vi "Tokens to Object.vi"(8 "error in":errorcluster, 10 "starting index":i32, 11 "array w/ subset deleted":cluster{"Token Type":T1, "Token Value":string}[](array[cluster])) -> (0 "error out":errorcluster, 2 "next index":i32, 3 "JSON Object out":refnum<class "JSON Object.lvclass">)   [LabVIEW 2017, in "LVJSON.lvlib"]
uses:
  LVJSON.lvlib
  JSON Data Classes/JSON Object/JSON Object.lvclass
  C:/Users/tblair/Documents/Git Projects/LVJSON/JSON Data Classes/JSON Datatype/JSON Datatype.lvclass
  Token Types.ctl
  JSON Data Classes/JSON Array/JSON Array.lvclass
  JSON Data Classes/JSON Numeric/JSON Numeric.lvclass
  JSON Data Classes/JSON Boolean/JSON Boolean.lvclass
  JSON Data Classes/JSON Null/JSON Null.lvclass
  JSON Data Classes/JSON String/JSON String.lvclass
  JSON Data Classes/JSON Numeric/New JSON Numeric.vi
  JSON Data Classes/JSON Boolean/New JSON Boolean.vi
  JSON Data Classes/JSON Null/New JSON Null.vi
  JSON Data Classes/JSON String/New JSON String.vi
  JSON Data Classes/JSON Object/New JSON Object.vi
  JSON Data Classes/JSON Object/Insert Key Value Pair (Multi).vi
  JSON Data Classes/JSON Datatype/JSON Datatype.lvclass
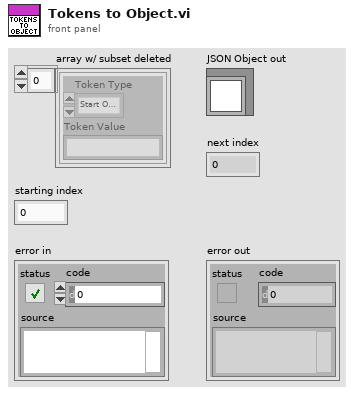
[diagram p1: front panel]
types:
  T1 = typedef "Token Types.ctl" = enum32{"Start Object", "End Object", "Start Array", "End Array", "Colon", "Comma", "Numeric", "true", "false", "null", "String"}
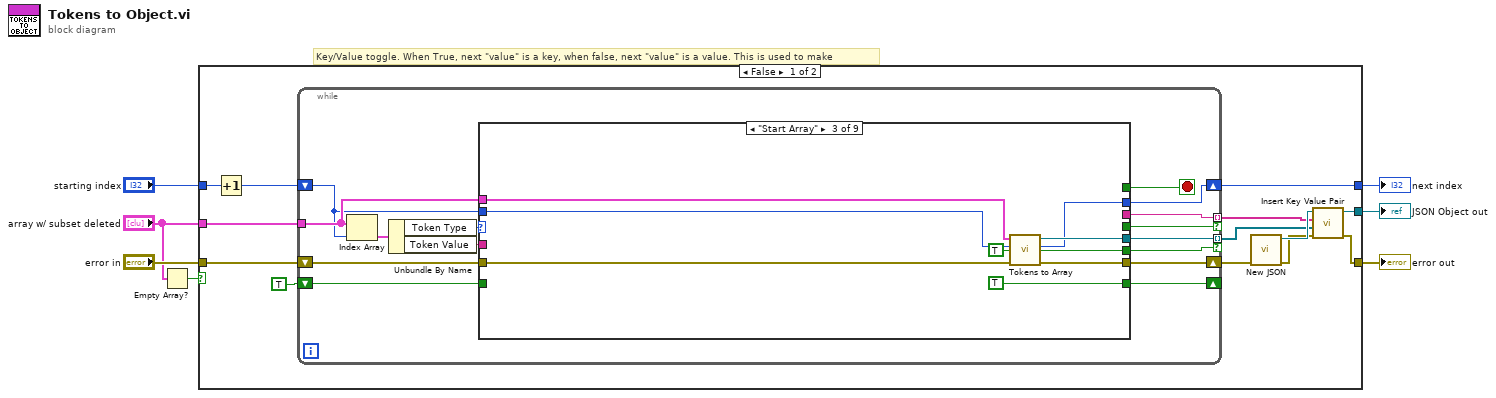
[diagram p0: block diagram]
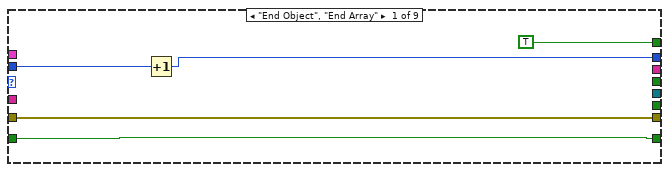
[diagram p2: hidden frame]
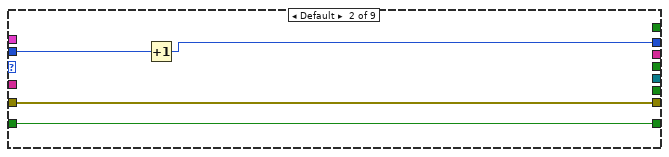
[diagram p3: hidden frame]
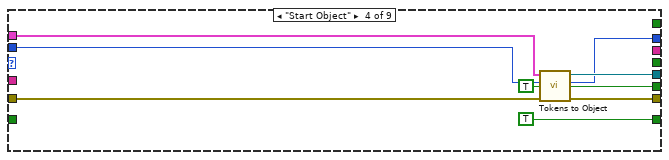
[diagram p4: hidden frame]
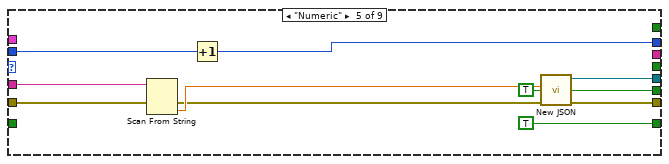
[diagram p5: hidden frame]
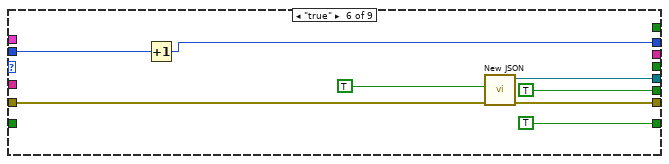
[diagram p6: hidden frame]
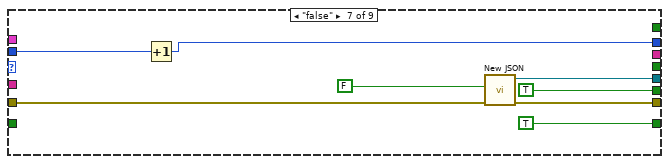
[diagram p7: hidden frame]
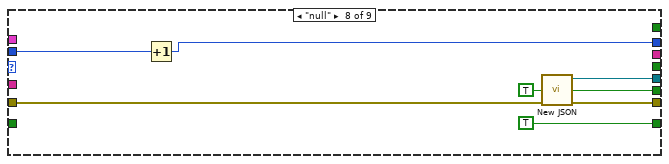
[diagram p8: hidden frame]
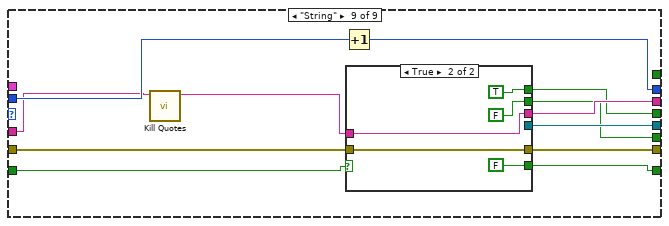
[diagram p9: hidden frame]
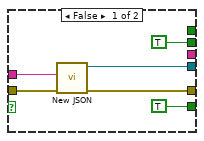
[diagram p10: hidden frame]
diagram:
  # "Key/Value toggle. When True, next \"value\" is a key, when false, next \"value\" is a value. This is used to make"
  n1 = Empty Array?(array="array w/ subset deleted") -> (empty?=w1:bool)
  n2 = case shown="False" w1 {
    tunnel: [w13 _] -> w7
    tunnel: "array w/ subset deleted" -> [w20 _]
    tunnel: "error in" -> [w19 w117]
    tunnel: [w8 w117] -> w5
    tunnel: [w16 w118] -> w4
    tunnel: "starting index" -> [w15 w118]
    frame False {
      n3 = Increment(x=w15) -> (x+1=w17:i32)
      n4 = while {
        tunnel: w20 -> [w28]
        tunnel: [w32] -> w12 mode=indexing if=w21
        shift-right: [w27] -> w16
        shift-left: w17 -> [w26]
        shift-right: [w29] -> w18
        shift-left: w19 -> [w30]
        shift-right: [w22] -> _
        shift-left: TRUE -> [w25]
        tunnel: [w24] -> w10 mode=indexing if=w23
        stop <- w33 stop-if-true
        n5 = Index Array(array=w28, index=w26) -> (element=w31:cluster{"Token Type":T1, "Token Value":string})
        n6 = Unbundle By Name(w31) -> ("Token Type"=w35:T1, "Token Value"=w34:string)
        n7 = case shown="\"Start Array\"" w35 {
          tunnel: w34 -> [_ _ _ _ w69 _ _ _ w94]
          tunnel: [TRUE _ _ _ _ _ _ _ _] -> w33
          tunnel: [_ _ w49 w57 w70 w77 w85 w93 w105] -> w32
          tunnel: [_ _ TRUE TRUE TRUE TRUE TRUE TRUE w97] -> w21
          tunnel: w30 -> [w40 w44 w52 w60 w66 w75 w83 w91 w96]
          tunnel: [w40 w44 w51 w59 w64 w74 w82 w90 w104] -> w29
          tunnel: w28 -> [_ _ w50 w58 _ _ _ _ _]
          tunnel: w26 -> [w39 w43 w46 w54 w63 w73 w81 w89 w103]
          tunnel: [w38 w42 w47 w55 w62 w72 w80 w88 w102] -> w27
          tunnel: w25 -> [w36 w41 _ _ _ _ _ _ w101]
          tunnel: [w36 w41 TRUE TRUE TRUE TRUE TRUE TRUE w98] -> w22
          tunnel: [_ _ _ _ _ _ _ _ w100] -> w24
          tunnel: [_ _ _ _ _ _ _ _ w99] -> w23
          frame "End Object", "End Array" {
            n8 = Increment(x=w39) -> (x+1=w38:i32)
          }
          frame Default {
            n9 = Increment(x=w43) -> (x+1=w42:i32)
          }
          frame "Start Array" {
            n10 = call "Tokens to Array.vi"("error in"=w52, "starting index"=w46, "array w/ subset deleted"=w50) -> ("error out"=w51:errorcluster, "next index"=w47:i32, "JSON Array out"=w49:refnum<class "JSON Array.lvclass">)  [unwired: 6 in]
          }
          frame "Start Object" {
            n11 = call "Tokens to Object.vi"("error in"=w60, "starting index"=w54, "array w/ subset deleted"=w58) -> ("error out"=w59:errorcluster, "next index"=w55:i32, "JSON Object out"=w57:refnum<class "JSON Object.lvclass">)  [unwired: 6 in]
          }
          frame "Numeric" {
            n12 = Scan From String(input string=w69, error in=w66) -> (error out=w65:errorcluster, output 1=w68:dbl)  [unwired: 3 in, 2 out]
            n13 = Increment(x=w63) -> (x+1=w62:i32)
            n14 = call-poly "New JSON.vi"("error in (no error)"=w65, "value"=w68) -> ("error out"=w64:errorcluster, "JSON String out"=w70:refnum<class "JSON Numeric.lvclass">)  [unwired: 8 in]
          }
          frame "true" {
            n15 = Increment(x=w73) -> (x+1=w72:i32)
            n16 = call-poly "New JSON.vi"("error in (no error)"=w75, "value"=TRUE) -> ("error out"=w74:errorcluster, "JSON String out"=w77:refnum<class "JSON Boolean.lvclass">)  [unwired: 8 in]
          }
          frame "false" {
            n17 = Increment(x=w81) -> (x+1=w80:i32)
            n18 = call-poly "New JSON.vi"("error in (no error)"=w83, "value"=FALSE) -> ("error out"=w82:errorcluster, "JSON String out"=w85:refnum<class "JSON Boolean.lvclass">)  [unwired: 8 in]
          }
          frame "null" {
            n19 = Increment(x=w89) -> (x+1=w88:i32)
            n20 = call-poly "New JSON.vi"("error in (no error)"=w91) -> ("error out"=w90:errorcluster, "JSON String out"=w93:refnum<class "JSON Null.lvclass">)  [unwired: 9 in]
          }
          frame "String" {
            n21 = call "Kill Quotes.vi"("Token Value in"=w94) -> ("Token Value out"=w95:string)  [unwired: 10 in]
            n22 = Increment(x=w103) -> (x+1=w102:i32)
            n23 = case shown="True" w101 {
              tunnel: [w111 _] -> w105
              tunnel: w95 -> [w110 w114]
              tunnel: w96 -> [w109 w115]
              tunnel: [w108 w115] -> w104
              tunnel: [TRUE FALSE] -> w97
              tunnel: [_ w114] -> w100
              tunnel: [_ TRUE] -> w99
              tunnel: [TRUE FALSE] -> w98
              frame False {
                n24 = call-poly "New JSON.vi"("error in (no error)"=w109, "value"=w110) -> ("error out"=w108:errorcluster, "JSON String out"=w111:refnum<class "JSON String.lvclass">)  [unwired: 8 in]
              }
              frame True {
              }
            }
          }
        }
      }
      n25 = call-poly "New JSON.vi"("error in (no error)"=w18) -> ("error out"=w9:errorcluster, "JSON Object out"=w14:refnum<class "JSON Object.lvclass">)  [unwired: 9 in]
      n26 = call-poly "Insert Key Value Pair.vi"("error in (no error)"=w9, "values"=w12, "keys"=w10, "JSON Object in"=w14) -> ("error out"=w8:errorcluster, "JSON Object out"=w13:refnum<class "JSON Object.lvclass">)  [unwired: 6 in]
    }
    frame True {
    }
  }
  "next index" <- w4
  "JSON Object out" <- w7
  "error out" <- w5
